vi "URL Generator.vi"(8 "error in (no error)":errorcluster, 10 "Append URL":string, 11 "API Command":T1) -> (0 "error out":errorcluster, 3 "Generated URL":string)   [LabVIEW 2014, in "FIRST Events API.lvlib"]
uses:
  FIRST Events API.lvlib
  FRC API Selector.ctl
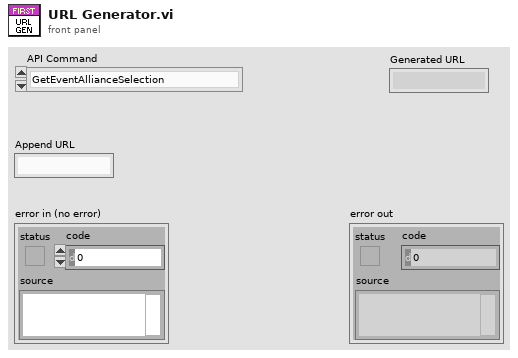
[diagram p1: front panel]
types:
  T1 = typedef "FIRST Events API.lvlib/FRC API Selector.ctl" = enum16{"GetEventAllianceSelection", "Ancillary", "GetTeamListings", "GetSchedule", "GetEventListings"}
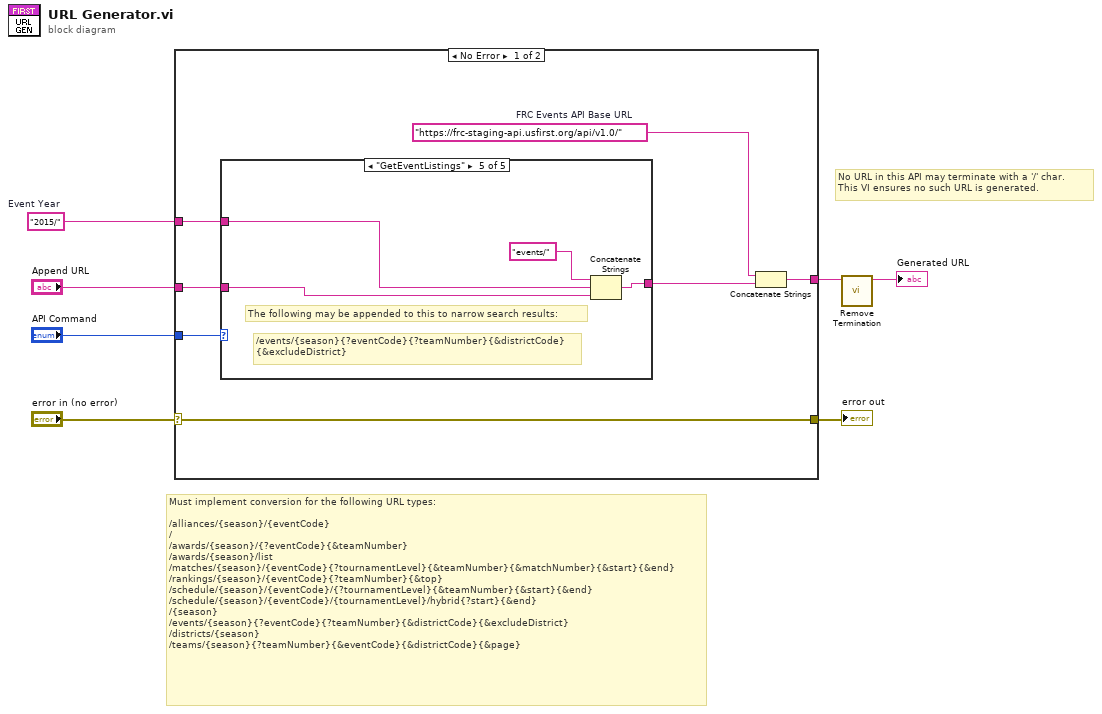
[diagram p0: block diagram]
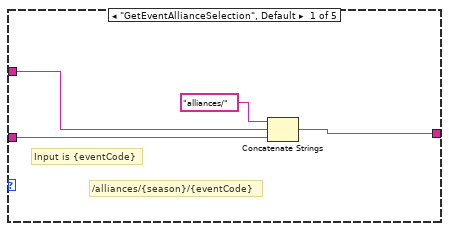
[diagram p2: hidden frame]
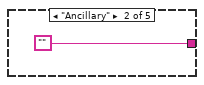
[diagram p3: hidden frame]
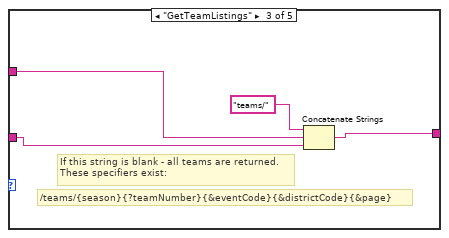
[diagram p4: hidden frame]
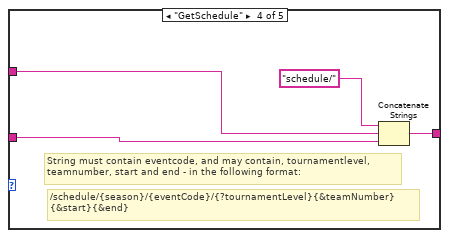
[diagram p5: hidden frame]
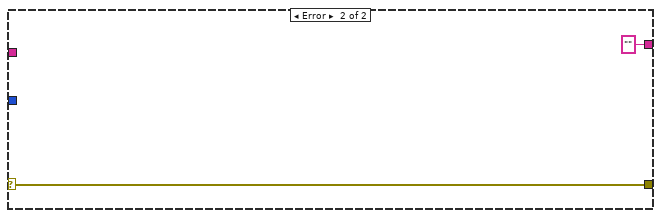
[diagram p6: hidden frame]
diagram:
  w6 = "2015/"  # Event Year
  # "No URL in this API may terminate with a '/' char.\nThis VI ensures no such URL is generated."
  # "Must implement conversion for the following URL types:\n\n/alliances/{season}/{eventCode}\n/\n/awards/{season}/{?eventCode}{&teamNumber}\n/awards/{season}/list\n/matches/{season}/{eventCode}{?tournamentLevel}{&teamNumber}{&matchNumber}{&start}{&end}\n/rankings/{season}/{eventCode}{?teamNumber}{&top}\n/schedule/{season}/{eventCode}/{?tournamentLevel}{&teamNumber}{&start}{&end}\n/schedule/{season}/{eventCode}/{tournamentLevel}/hybrid{?start}{&end}\n/{season}\n/events/{season}{?eventCode}{?teamNumber}{&districtCode}{&excludeDistrict}\n/districts/{season}\n/teams/{season}{?teamNumber}{&eventCode}{&districtCode}{&page}"
  n1 = case shown="No Error" "error in (no error)" {
    selector: "error in (no error)" -> [w8 w32]
    tunnel: "API Command" -> [w13 _]
    tunnel: w6 -> [w12 _]
    tunnel: "Append URL" -> [w11 _]
    tunnel: [w9 ""] -> w2
    tunnel: [w8 w32] -> w3
    frame No Error {
      w14 = "https://frc-staging-api.usfirst.org/api/v1.0/"  # FRC Events API Base URL
      n2 = case shown="\"GetEventListings\"" w13 {
        tunnel: w12 -> [w18 _ w20 w25 w29]
        tunnel: w11 -> [w17 _ w21 w24 w28]
        tunnel: [w16 "" w23 w27 w31] -> w10
        frame "GetEventAllianceSelection", Default {
          # "/alliances/{season}/{eventCode}"
          # "Input is {eventCode}"
          n3 = Concatenate Strings("alliances/" ("string"), w18, w17) -> (w16:string)
        }
        frame "Ancillary" {
        }
        frame "GetTeamListings" {
          # "/teams/{season}{?teamNumber}{&eventCode}{&districtCode}{&page}"
          # "If this string is blank - all teams are returned.\nThese specifiers exist:"
          n4 = Concatenate Strings("teams/" ("string"), w20, w21) -> (w23:string)
        }
        frame "GetSchedule" {
          # "/schedule/{season}/{eventCode}/{?tournamentLevel}{&teamNumber}\n{&start}{&end}"
          # "String must contain eventcode, and may contain, tournamentlevel,\nteamnumber, start and end - in the following format:"
          n5 = Concatenate Strings("schedule/" ("string"), w25, w24) -> (w27:string)
        }
        frame "GetEventListings" {
          # "/events/{season}{?eventCode}{?teamNumber}{&districtCode}\n{&excludeDistrict}"
          # "The following may be appended to this to narrow search results:"
          n6 = Concatenate Strings("events/" ("string"), w29, w28) -> (w31:string)
        }
      }
      n7 = Concatenate Strings(w14, w10) -> (w9:string)
    }
    frame Error {
    }
  }
  "error out" <- w3
  n8 = call "Remove Termination.vi"("String"=w2) -> ("substring"=→"Generated URL":string)  [unwired: 10 in]
